vi "random stuff.vi"   [LabVIEW 2012]
uses:
  Class/LV Wiimote Interface.lvclass
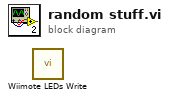
[diagram p0: block diagram]
diagram:
  n1 = call "Wiimote LEDs Write.vi"() -> ()  [unwired: 9 in, 3 out]
